vi "GetMDT69Value.vi"(8 "error in (no error)":errorcluster, 10 "Channel":string, 11 "VISA resource name":refnum<visa-resource-name>) -> (0 "error out":errorcluster, 2 "Value":string, 3 "VISA resource name":refnum<visa-resource-name>)   [LabVIEW 2020]
uses:
  Match Regular Expression.xnode
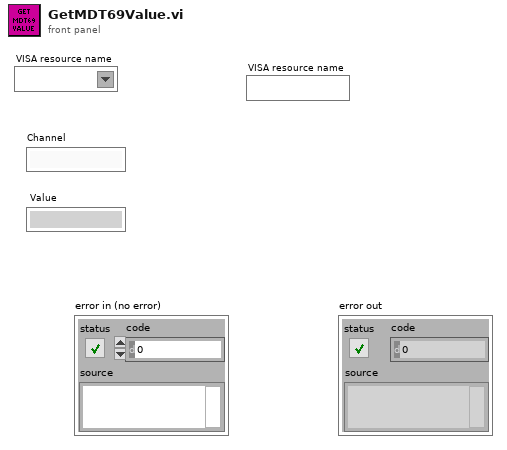
[diagram p1: front panel]
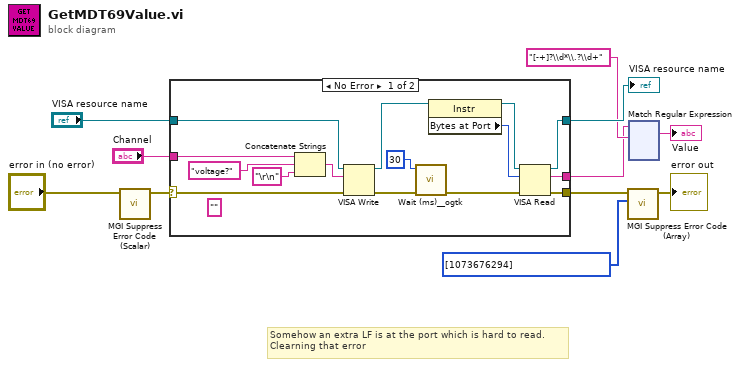
[diagram p0: block diagram]
diagram:
  # "Somehow an extra LF is at the port which is hard to read.\nClearning that error"
  n1 = call "MGI Suppress Error Code (Scalar).vi"("Error In"="error in (no error)") -> ("Error Out"=w4:errorcluster)  [unwired: 5 in, 1 out]
  n2 = case shown="No Error" w4 {
    selector: w4 -> [w22 w28]
    tunnel: [w13 w28] -> w3
    tunnel: "VISA resource name" -> [w23 w27]
    tunnel: [w12 w27] -> w10
    tunnel: "Channel" -> [w26 _]
    tunnel: [w17 _] -> w6
    frame No Error {
      (unwired) ""
      n3 = Concatenate Strings(w26, "voltage?" ("string"), "\r\n" ("string")) -> (w24:string)
      n4 = VISA Write(VISA resource name=w23, write buffer=w24, error in (no error)=w22) -> (VISA resource name out=w16:refnum<visa-resource-name>, error out=w20:errorcluster)  [unwired: 1 out]
      n5 = call "Wait (ms)__ogtk.vi"("error in (no error)"=w20, "milliseconds to wait"=u32 30) -> ("error out"=w18:errorcluster)  [unwired: 8 in, 1 out]
      n6 = property class="Instr"(reference=w16) -> (reference out=w15:refnum<visa-resource-name>, "Bytes at Port"=w14:u32)  [unwired: 1 in, 1 out]
      n7 = VISA Read(VISA resource name=w15, byte count=w14, error in (no error)=w18) -> (VISA resource name out=w12:refnum<visa-resource-name>, read buffer=w17:string, error out=w13:errorcluster)  [unwired: 1 out]
    }
    frame Error {
    }
  }
  "VISA resource name" <- w10
  n8 = call "MGI Suppress Error Code (Array).vi"("Error Codes[]"=i32[] [1073676294] ("Error Codes to Filter"), "Error In"=w3) -> ("Error Out"=→"error out":errorcluster)  [unwired: 4 in, 1 out]
  n9 = xnode "Match Regular Expression"("input string"=w6, "regular expression"="[-+]?\\d*\\.?\\d+") -> ("whole match"=→"Value":string)  [unwired: 4 in, 4 out]
